vi "WS105x Bench Single Socket Package Test Program Ver1.0.vi"() -> ()   [LabVIEW 2012]
uses:
  SubVI/Type Def/WS1050 Test Sequences.ctl
  <instrlib>/Tektronix DPO MSO 2000 4000 Series/Tektronix DPO MSO 2000 4000 Series.lvlib
panel:
  in  "Tab Control":enum32{"Control", "Indicator"}(tab)
  out "Sequence":i32(listbox)=5
  in  "Header Table":string[][](table)=[["Lot#", "Wafer#", "SN#", "", "", "", "", "", "I_total"], ["WS1050", "T7", "1", "", "", "", "", "", "0.000000E+0"]]
  in  "TMN DC\\CAP Data Log File Path":path=path "C:/Andy/WS1050/Full TP/Multi VPI"
  in  "Title":string="WS105x_Bench_Single Socket_Package Test Program Ver1.0"
  in  "Equipment":T1={"Dev 6501"="Dev2/port2/line0", "CAP Meas "="COM8", "A364X_VDD"="GPIB1::6::INSTR", "Ke2400_VSA"="GPIB1::1::INSTR", "Ke2000_IDD"="GPIB1::9::INSTR", "RFFE"="COM3", "Scope USB"="USB0::0x0699::0x0405::C010240::INSTR"}
  in  "START \nTEST":bool
  in  "stop":bool
  out "1050 Test Sequences":T2
  in  "IDD Limit":dbl=0.02 format="%.2p"
  out "error out":errorcluster
  in  "error in (no error)":errorcluster
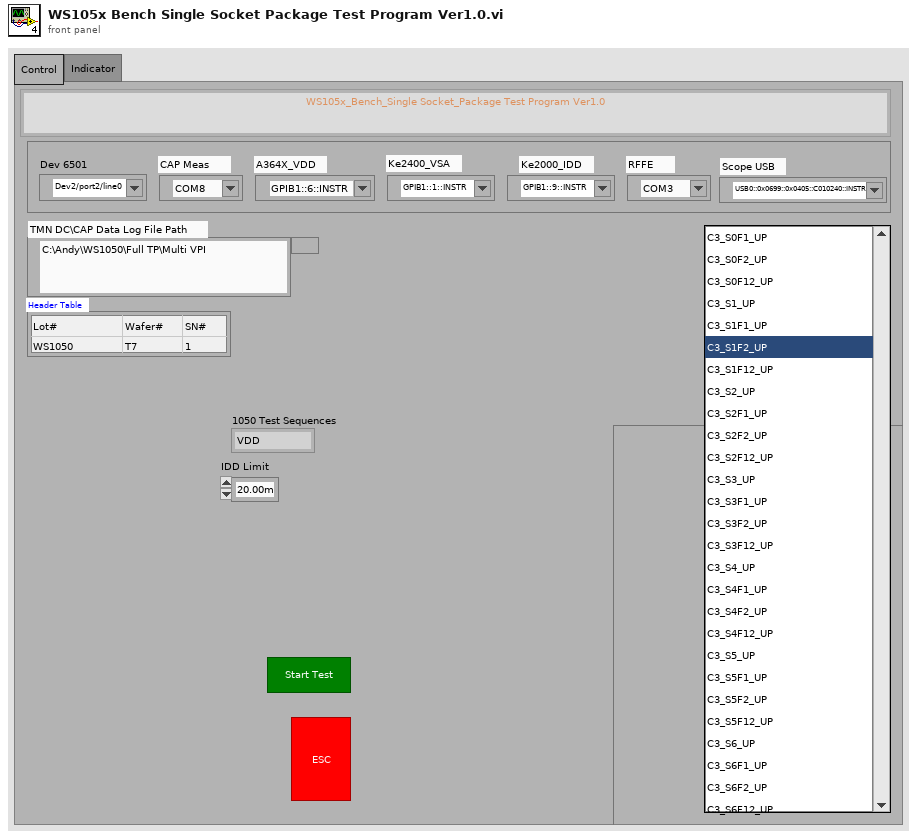
[diagram p1: front panel]
types:
  T1 = cluster{"Dev 6501":tag, "CAP Meas ":refnum<visa-resource-name>, "A364X_VDD":refnum<visa-resource-name>, "Ke2400_VSA":refnum<visa-resource-name>, "Ke2000_IDD":refnum<visa-resource-name>, "RFFE":refnum<visa-resource-name>, "Scope USB":refnum<visa-resource-name>}
  T2 = typedef "WS1050 Test Sequences.ctl" = enum16{"VDD", "Toggle CP", "Test Cond", "IDD Meas", "Cap Meas", "VPI", "VSA", "ST", "Save Data", "Exit"}
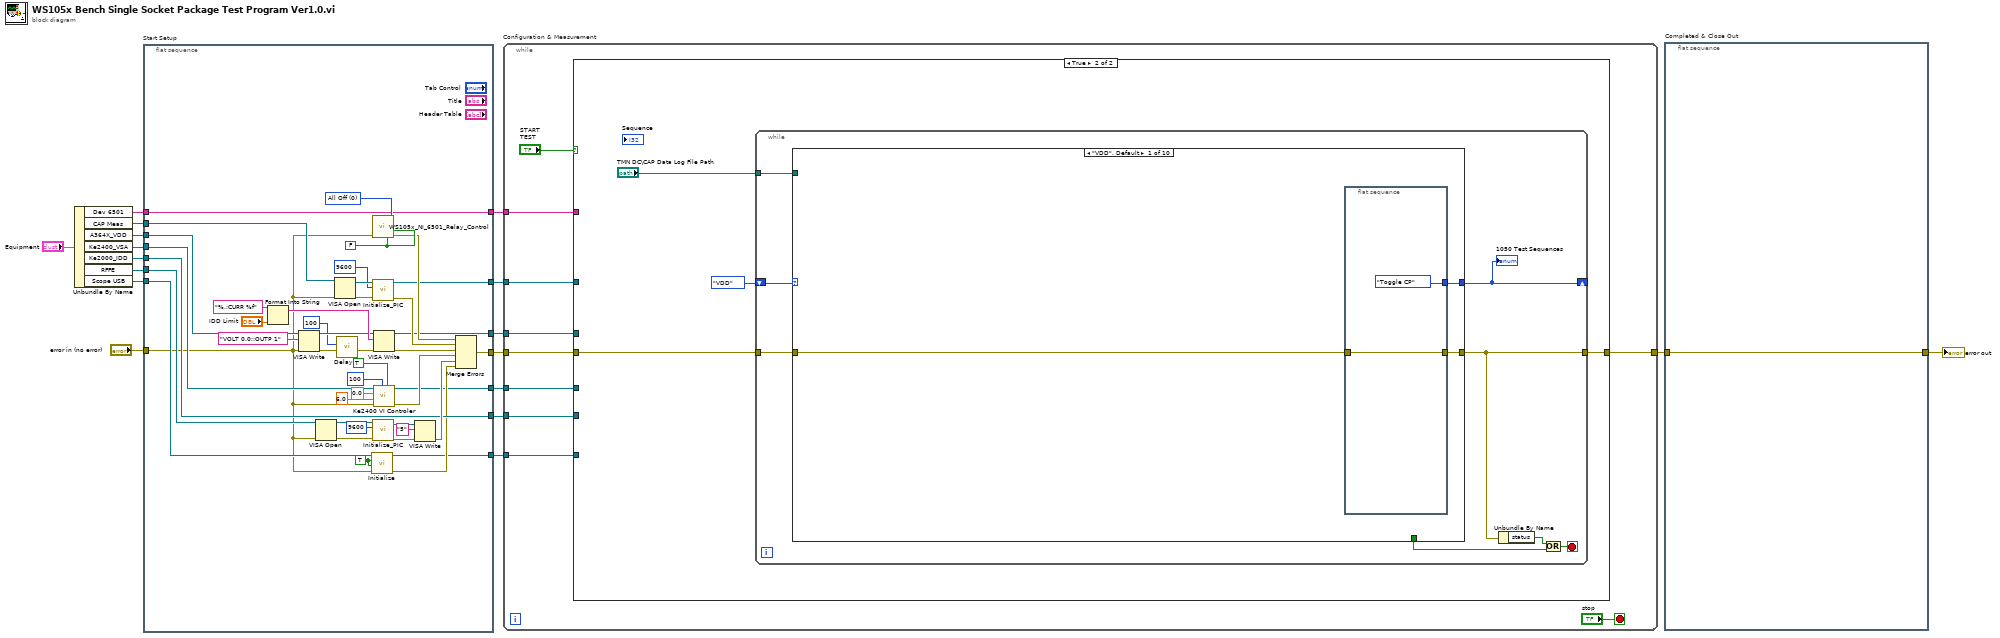
[diagram p0: block diagram]
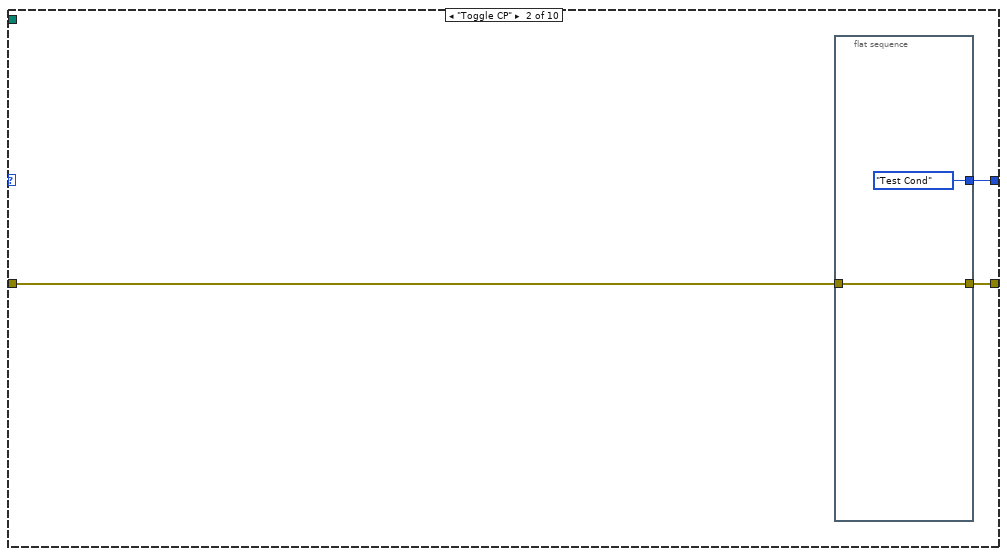
[diagram p3: hidden frame]
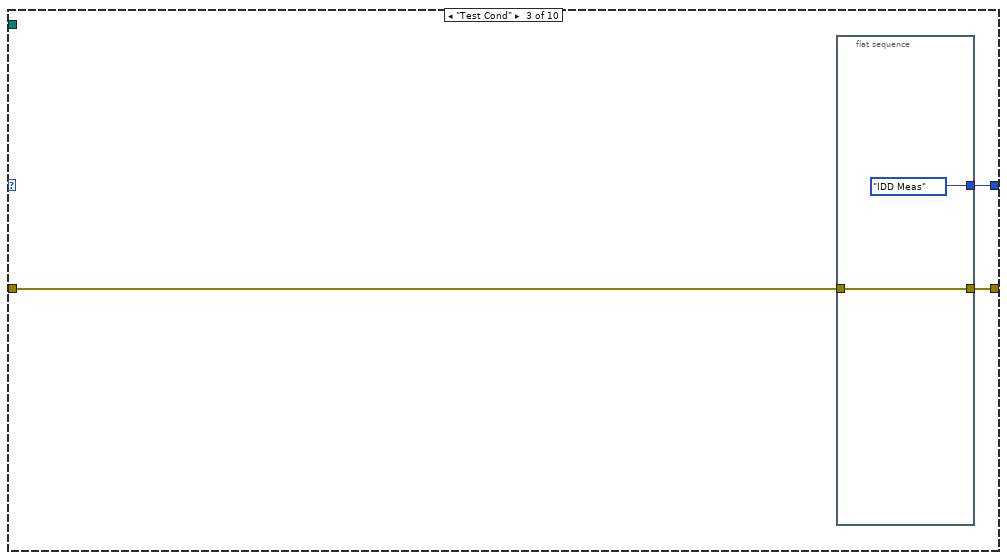
[diagram p4: hidden frame]
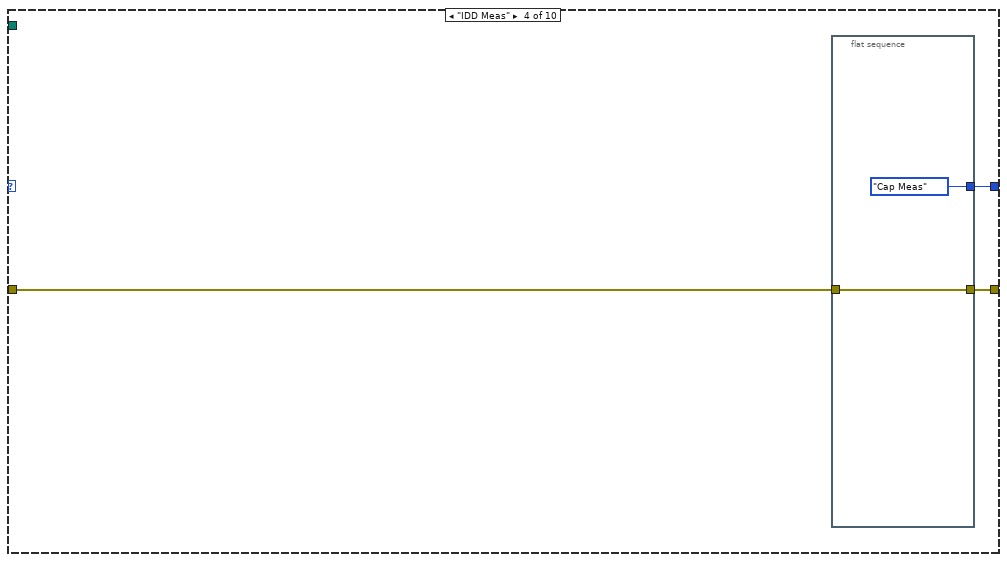
[diagram p5: hidden frame]
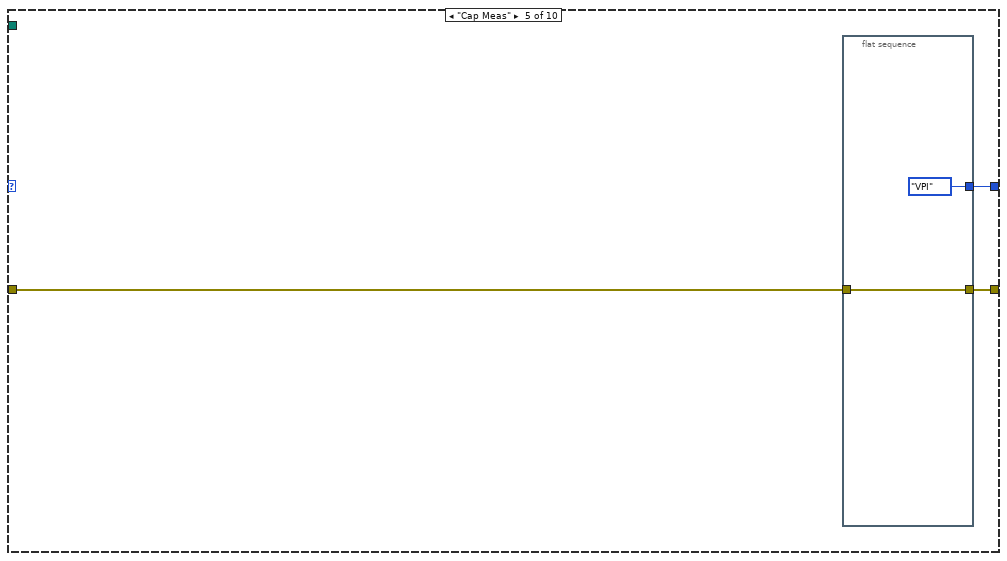
[diagram p6: hidden frame]
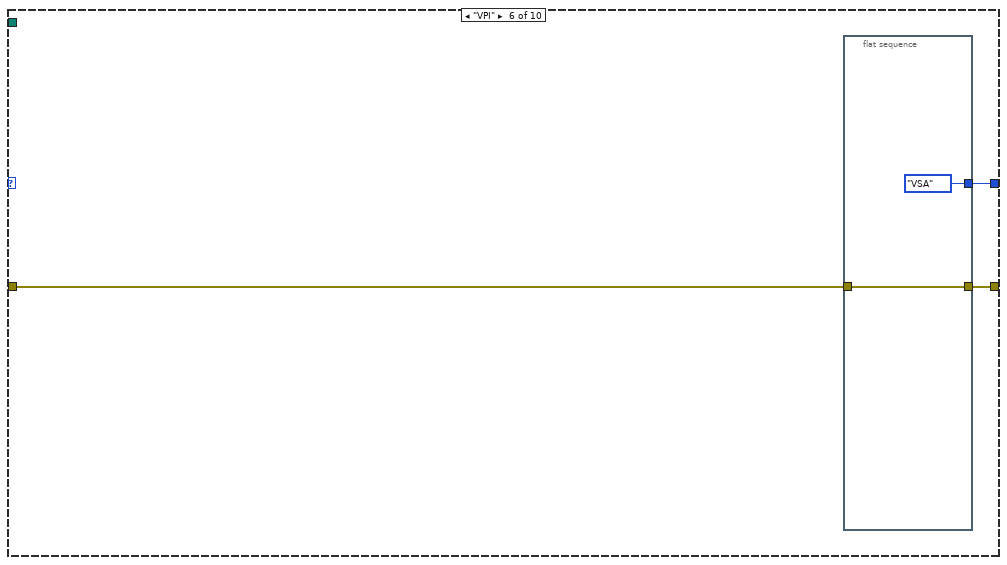
[diagram p7: hidden frame]
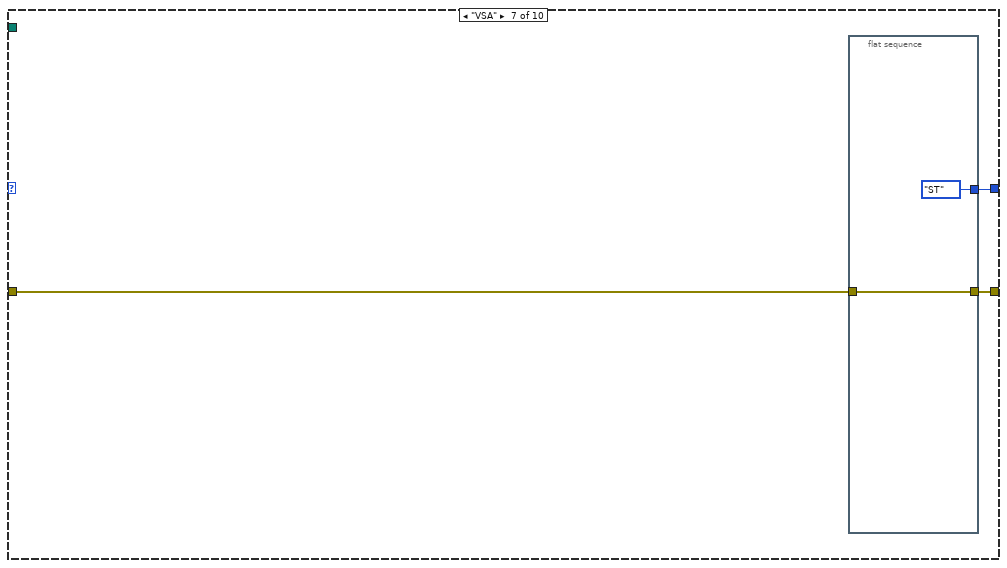
[diagram p8: hidden frame]
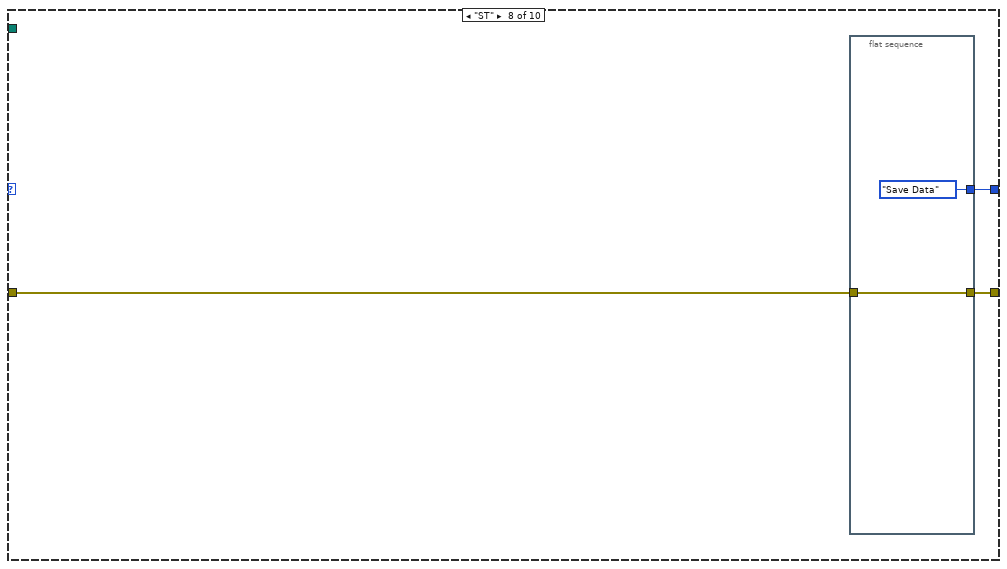
[diagram p9: hidden frame]
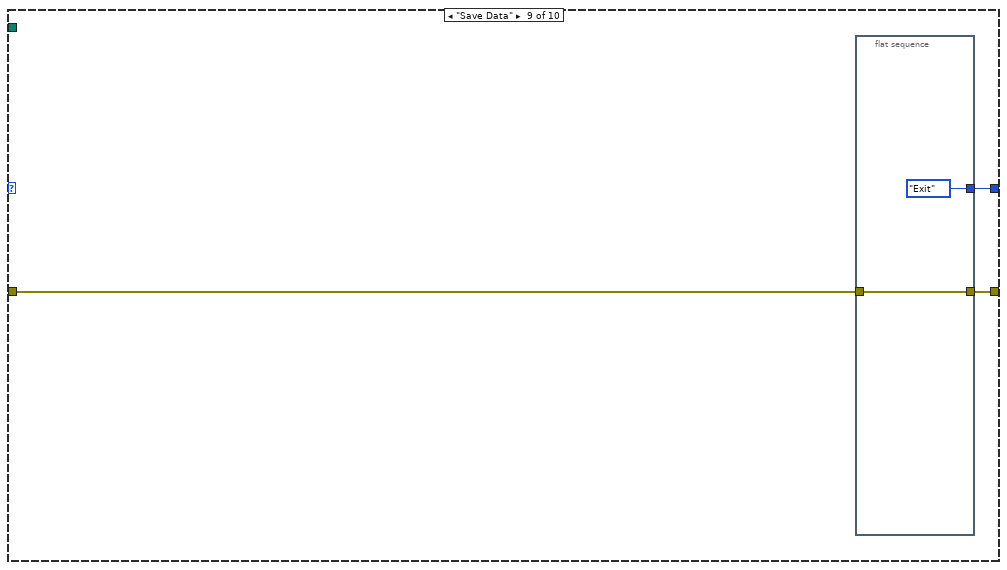
[diagram p10: hidden frame]
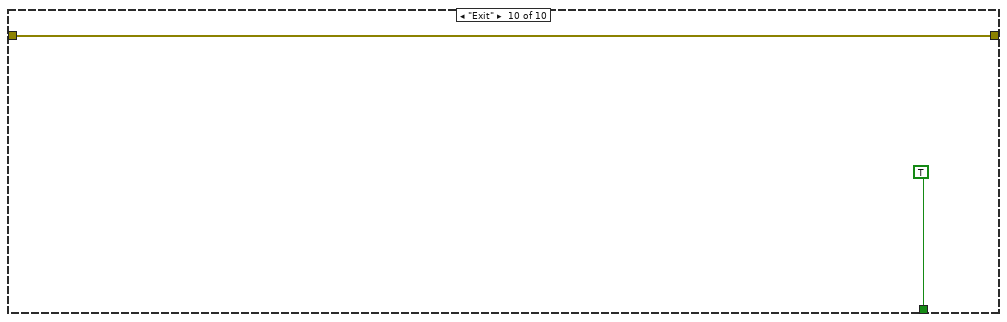
[diagram p11: hidden frame]
diagram:
  n1 = Unbundle By Name("Equipment") -> ("Dev 6501"=w15:tag, "CAP Meas"=w14:refnum<visa-resource-name>, "A364X_VDD"=w13:refnum<visa-resource-name>, "Ke2400_VSA"=w12:refnum<visa-resource-name>, "Ke2000_IDD"=w11:refnum<visa-resource-name>, "RFFE"=w10:refnum<visa-resource-name>, "Scope USB"=w9:refnum<visa-resource-name>)
  n2 = flat-sequence "Start Setup" {
    tunnel: [w29] -> w18
    tunnel: w15 -> [w26]
    tunnel: w14 -> [w35]
    tunnel: w13 -> [w34]
    tunnel: w12 -> [w33]
    tunnel: w11 -> [w31]
    tunnel: w10 -> [w32]
    tunnel: [w31] -> w5
    tunnel: w9 -> [w30]
    tunnel: "error in (no error)" -> [w28]
    tunnel: [w26] -> w7
    tunnel: [w25] -> w6
    tunnel: [w24] -> w4
    tunnel: [w23] -> w3
    tunnel: [w22] -> w2
    frame #0 {
      w61 = TRUE ("ID Query")
      w59 = FALSE ("Relay_ 10")
      w58 = u16 0 items=["All Off", "Bank 1", "Bank 2", "Bank 3"] ("Ring")
      n3 = Format Into String(format string="%.;CURR %f", "IDD Limit") -> (resulting string=w44:string)  [unwired: 2 in, 1 out]
      n4 = VISA Write(VISA resource name=w34, write buffer="VOLT 0.0;:OUTP 1", error in (no error)=w28) -> (VISA resource name out=w43:refnum<visa-resource-name>, error out=w20:errorcluster)  [unwired: 1 out]
      n5 = VISA Open(error in (no error)=w28, VISA resource name=w32) -> (VISA resource name=w54:refnum<visa-resource-name>, error out=w53:errorcluster)  [unwired: 3 in]
      n6 = VISA Open(error in (no error)=w28, VISA resource name=w35) -> (VISA resource name=w56:refnum<visa-resource-name>, error out=w57:errorcluster)  [unwired: 3 in]
      n7 = call "Delay.vi"("error in (no error)"=w20, "milliseconds to wait"=u32 100) -> ("error out"=w21:errorcluster)  [unwired: 9 in]
      n8 = call <instrlib>:"Initialize.vi"("error in (no error)"=w28, "Reset (True)"=w61, "ID Query (True)"=w61, "VISA resource name"=w30) -> ("error out"=w27:errorcluster, "VISA resource name out"=w24:refnum<visa-resource-name>)  [unwired: 6 in]
      n9 = call "WS105x_NI_6501_Relay_Control.vi"("Ring"=w58, "Relay_ 11"=w59, "error in (no error)"=w28, "Relay_ 10"=w59) -> ("error out"=w36:errorcluster)  [unwired: 2 in, 9 out]
      n10 = call "Initialize_PIC.vi"("error in (no error)"=w57, "baud rate"=u32 9600, "Select Com Port"=w56) -> ("error out"=w48:errorcluster, "VISA resource name out"=w25:refnum<visa-resource-name>)  [unwired: 7 in]
      n11 = call "Initialize_PIC.vi"("error in (no error)"=w53, "baud rate"=u32 9600, "Select Com Port"=w54) -> ("error out"=w52:errorcluster, "VISA resource name out"=w51:refnum<visa-resource-name>)  [unwired: 7 in]
      n12 = VISA Write(VISA resource name=w43, write buffer=w44, error in (no error)=w21) -> (VISA resource name out=w23:refnum<visa-resource-name>, error out=w42:errorcluster)  [unwired: 1 out]
      n13 = call "Ke2400 VI Controler.vi"("ON/OFF"=TRUE, "Voltage Range"=100 ("Voltage Range(V)"), "error in (no error)"=w28, "Idd Compliace(mA)"=6.0 ("Current Compliance(mA)"), "Volt Level"=0.0 ("Volt Level(V)"), "VISA In"=w33) -> ("error out"=w41:errorcluster, "VISA Out"=w22:refnum<visa-resource-name>)  [unwired: 4 in]
      n14 = VISA Write(VISA resource name=w51, write buffer="5", error in (no error)=w52) -> (error out=w60:errorcluster)  [unwired: 2 out]
      n15 = Merge Errors(w36, w48, w42, w41, w60, w27) -> (w29:errorcluster)
    }
  }
  n16 = while "Configuration & Measurement" {
    tunnel: w18 -> [w69]
    tunnel: [w68] -> w17
    tunnel: w7 -> [w67]
    tunnel: w6 -> [w66]
    tunnel: w5 -> [w64]
    tunnel: w4 -> [w63]
    tunnel: w3 -> [w65]
    tunnel: w2 -> [w62]
    stop <- "stop" stop-if-true
    n17 = case shown="True" "START \nTEST" {
      tunnel: w69 -> [w72 w75]
      tunnel: [w72 w74] -> w68
      tunnel: w67 -> [_ _]
      tunnel: w66 -> [_ _]
      tunnel: w65 -> [_ _]
      tunnel: w64 -> [_ _]
      tunnel: w63 -> [_ _]
      tunnel: w62 -> [_ _]
      frame False {
      }
      frame True {
        n18 = while {
          tunnel: w75 -> [w83]
          tunnel: [w82] -> w74
          shift-right: [w81] -> _
          shift-left: WS1050_Test_Sequences."VDD" ("1050 Test Sequences") -> [w84]
          tunnel: "TMN DC\\CAP Data Log File Path" -> [w77]
          stop <- w80 stop-if-true
          n19 = case shown="\"VDD\", Default" w84 {
            tunnel: w83 -> [w87 w92 w96 w102 w107 w112 w117 w121 w126 w131]
            tunnel: [w85 w91 w95 w101 w106 w111 w116 w120 w125 w131] -> w82
            tunnel: [w86 w90 w97 w100 w105 w110 w115 w122 w127 _] -> w81
            tunnel: [_ _ _ _ _ _ _ _ _ TRUE] -> w78
            tunnel: w77 -> [_ _ _ _ _ _ _ _ _ _]
            frame "VDD", Default {
              n20 = flat-sequence {
                tunnel: w87 -> [w88]
                tunnel: [WS1050_Test_Sequences."Toggle CP" ("1050 Test Sequences")] -> w86
                tunnel: [w88] -> w85
                frame #0 {
                }
              }
            }
            frame "Toggle CP" {
              n21 = flat-sequence {
                tunnel: [w94] -> w91
                tunnel: w92 -> [w94]
                tunnel: [WS1050_Test_Sequences."Test Cond" ("1050 Test Sequences")] -> w90
                frame #0 {
                }
              }
            }
            frame "Test Cond" {
              n22 = flat-sequence {
                tunnel: [WS1050_Test_Sequences."IDD Meas" ("1050 Test Sequences")] -> w97
                tunnel: [w98] -> w95
                tunnel: w96 -> [w98]
                frame #0 {
                }
              }
            }
            frame "IDD Meas" {
              n23 = flat-sequence {
                tunnel: [w104] -> w101
                tunnel: w102 -> [w104]
                tunnel: [WS1050_Test_Sequences."Cap Meas" ("1050 Test Sequences")] -> w100
                frame #0 {
                }
              }
            }
            frame "Cap Meas" {
              n24 = flat-sequence {
                tunnel: [w109] -> w106
                tunnel: w107 -> [w109]
                tunnel: [WS1050_Test_Sequences."VPI" ("1050 Test Sequences")] -> w105
                frame #0 {
                }
              }
            }
            frame "VPI" {
              n25 = flat-sequence {
                tunnel: [w114] -> w111
                tunnel: w112 -> [w114]
                tunnel: [WS1050_Test_Sequences."VSA" ("1050 Test Sequences")] -> w110
                frame #0 {
                }
              }
            }
            frame "VSA" {
              n26 = flat-sequence {
                tunnel: [w119] -> w116
                tunnel: w117 -> [w119]
                tunnel: [WS1050_Test_Sequences."ST" ("1050 Test Sequences")] -> w115
                frame #0 {
                }
              }
            }
            frame "ST" {
              n27 = flat-sequence {
                tunnel: [WS1050_Test_Sequences."Save Data" ("1050 Test Sequences")] -> w122
                tunnel: [w123] -> w120
                tunnel: w121 -> [w123]
                frame #0 {
                }
              }
            }
            frame "Save Data" {
              n28 = flat-sequence {
                tunnel: [WS1050_Test_Sequences."Exit" ("1050 Test Sequences")] -> w127
                tunnel: [w128] -> w125
                tunnel: w126 -> [w128]
                frame #0 {
                }
              }
            }
            frame "Exit" {
            }
          }
          "1050 Test Sequences" <- w81
          n29 = Unbundle By Name(w82) -> ("status"=w79:bool)
          n30 = Or(x=w79, y=w78) -> (x .or. y?=w80:bool)
        }
      }
    }
  }
  n31 = flat-sequence "Completed & Close Out" {
    tunnel: w17 -> [w132]
    tunnel: [w132] -> w1
    frame #0 {
    }
  }
  "error out" <- w1
